vi "Imager_2.2.vi"() -> ()   [LabVIEW 2015]
doc: "You can repeat commands using for loop or while loop structures. This example shows how to use a for loop to replace the five <code>Move Relative -10000</code> commands in the previous example.\nNote that the error line needs to use a shift register in the loop, so that an error will get carried forward through later iterations.\nNow that you've seen two, here are some features common to most of our examples:\n* Place error and COM port wires in a straight line across the bottom. This is the main data flow of the diagram.\n* Start with Initialize to set timeouts and other things, and end with Close. If you don't use Close, Labview won't complain but other applications won't be able to use the COM port."
uses:
  <vilib>/Utility/config.llb/Write Key (I32).vi
  <vilib>/Utility/config.llb/Write Key (Path).vi
  <vilib>/Utility/config.llb/Write Key (String).vi
  <vilib>/Utility/config.llb/Write Key (U32).vi
  <vilib>/Utility/config.llb/Read Key (I32).vi
  <vilib>/Utility/config.llb/Read Key (Path).vi
  <vilib>/Utility/config.llb/Read Key (String).vi
  <vilib>/Utility/config.llb/NI_LVConfig.lvlib
panel:
  in  "Return home":bool
  in  "Reset Home":bool
  out "Move completed":bool
  out "Progress":string="\r\n"
  out "Image 2":T1(plugin-control)
  out "Current Plate 2":dbl
  in  "Plate Diameter (steps) 2":i32=5000
  in  "Live":bool
  in  "start path for config files":path=path "C:/images" caption="start path"
  in  "Load Settings":bool
  in  "Settings":bool
  in  "Offset to Plate 1 (steps)":i32=4000
  in  "Camera ID":u32=285941632
  in  "Pause (s)":u32
  out "Current Plate":dbl
  in  "Total Number of plates":i32=14 min=2
  out "plate number":i32
  out "Next plate number":i32
  out "first plate number":dbl
  out "Run":dbl
  in  "?":bool
  in  "EXIT":bool
  in  "Clear Settings":bool
  in  "START":bool
  in  "Plate Diameter (steps)":i32=5200
  out "Pause (seconds)":u32
  in  "Save Path":path=path "C:/images"
  in  "Port":refnum<visa-resource-name>="COM3"
  # "Plate Imager V2.0"
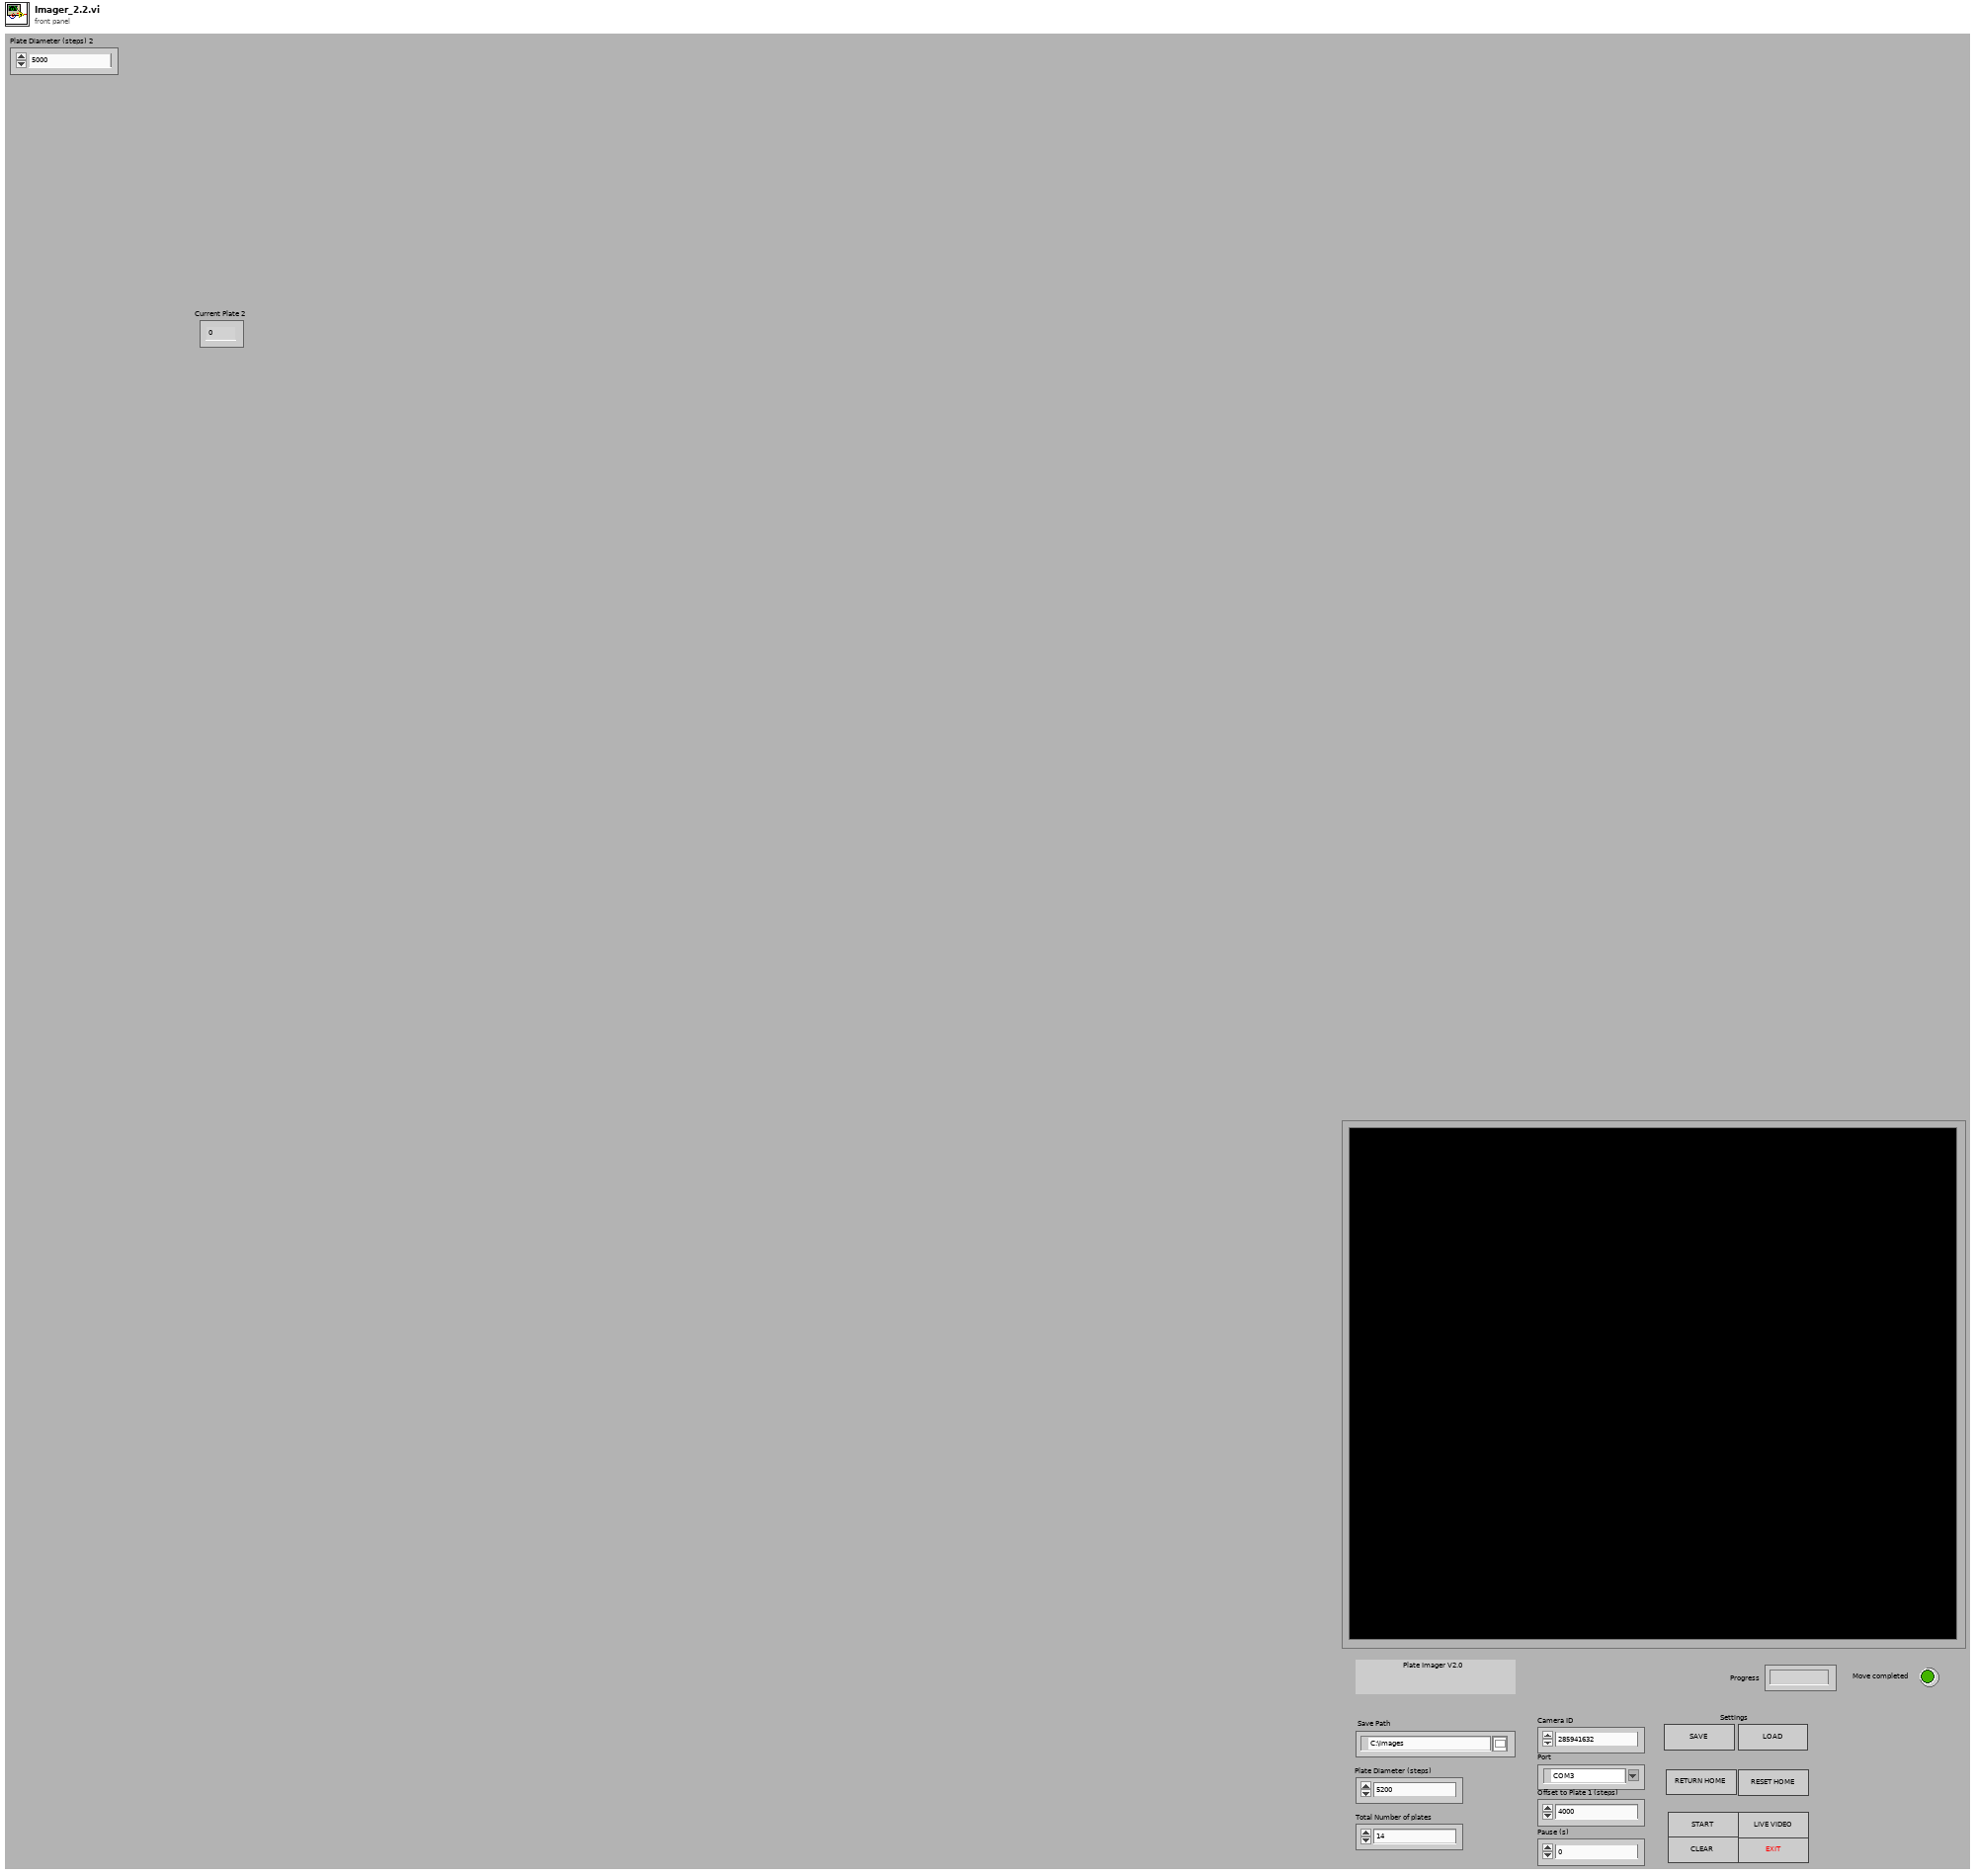
[diagram p1: front panel]
types:
  T1 = typedef "IMAQ Image.ctl" = refnum<image>
  T2 = typedef "NI_LVConfig.lvlib/Config Data RefNum.ctl" = refnum<k1>
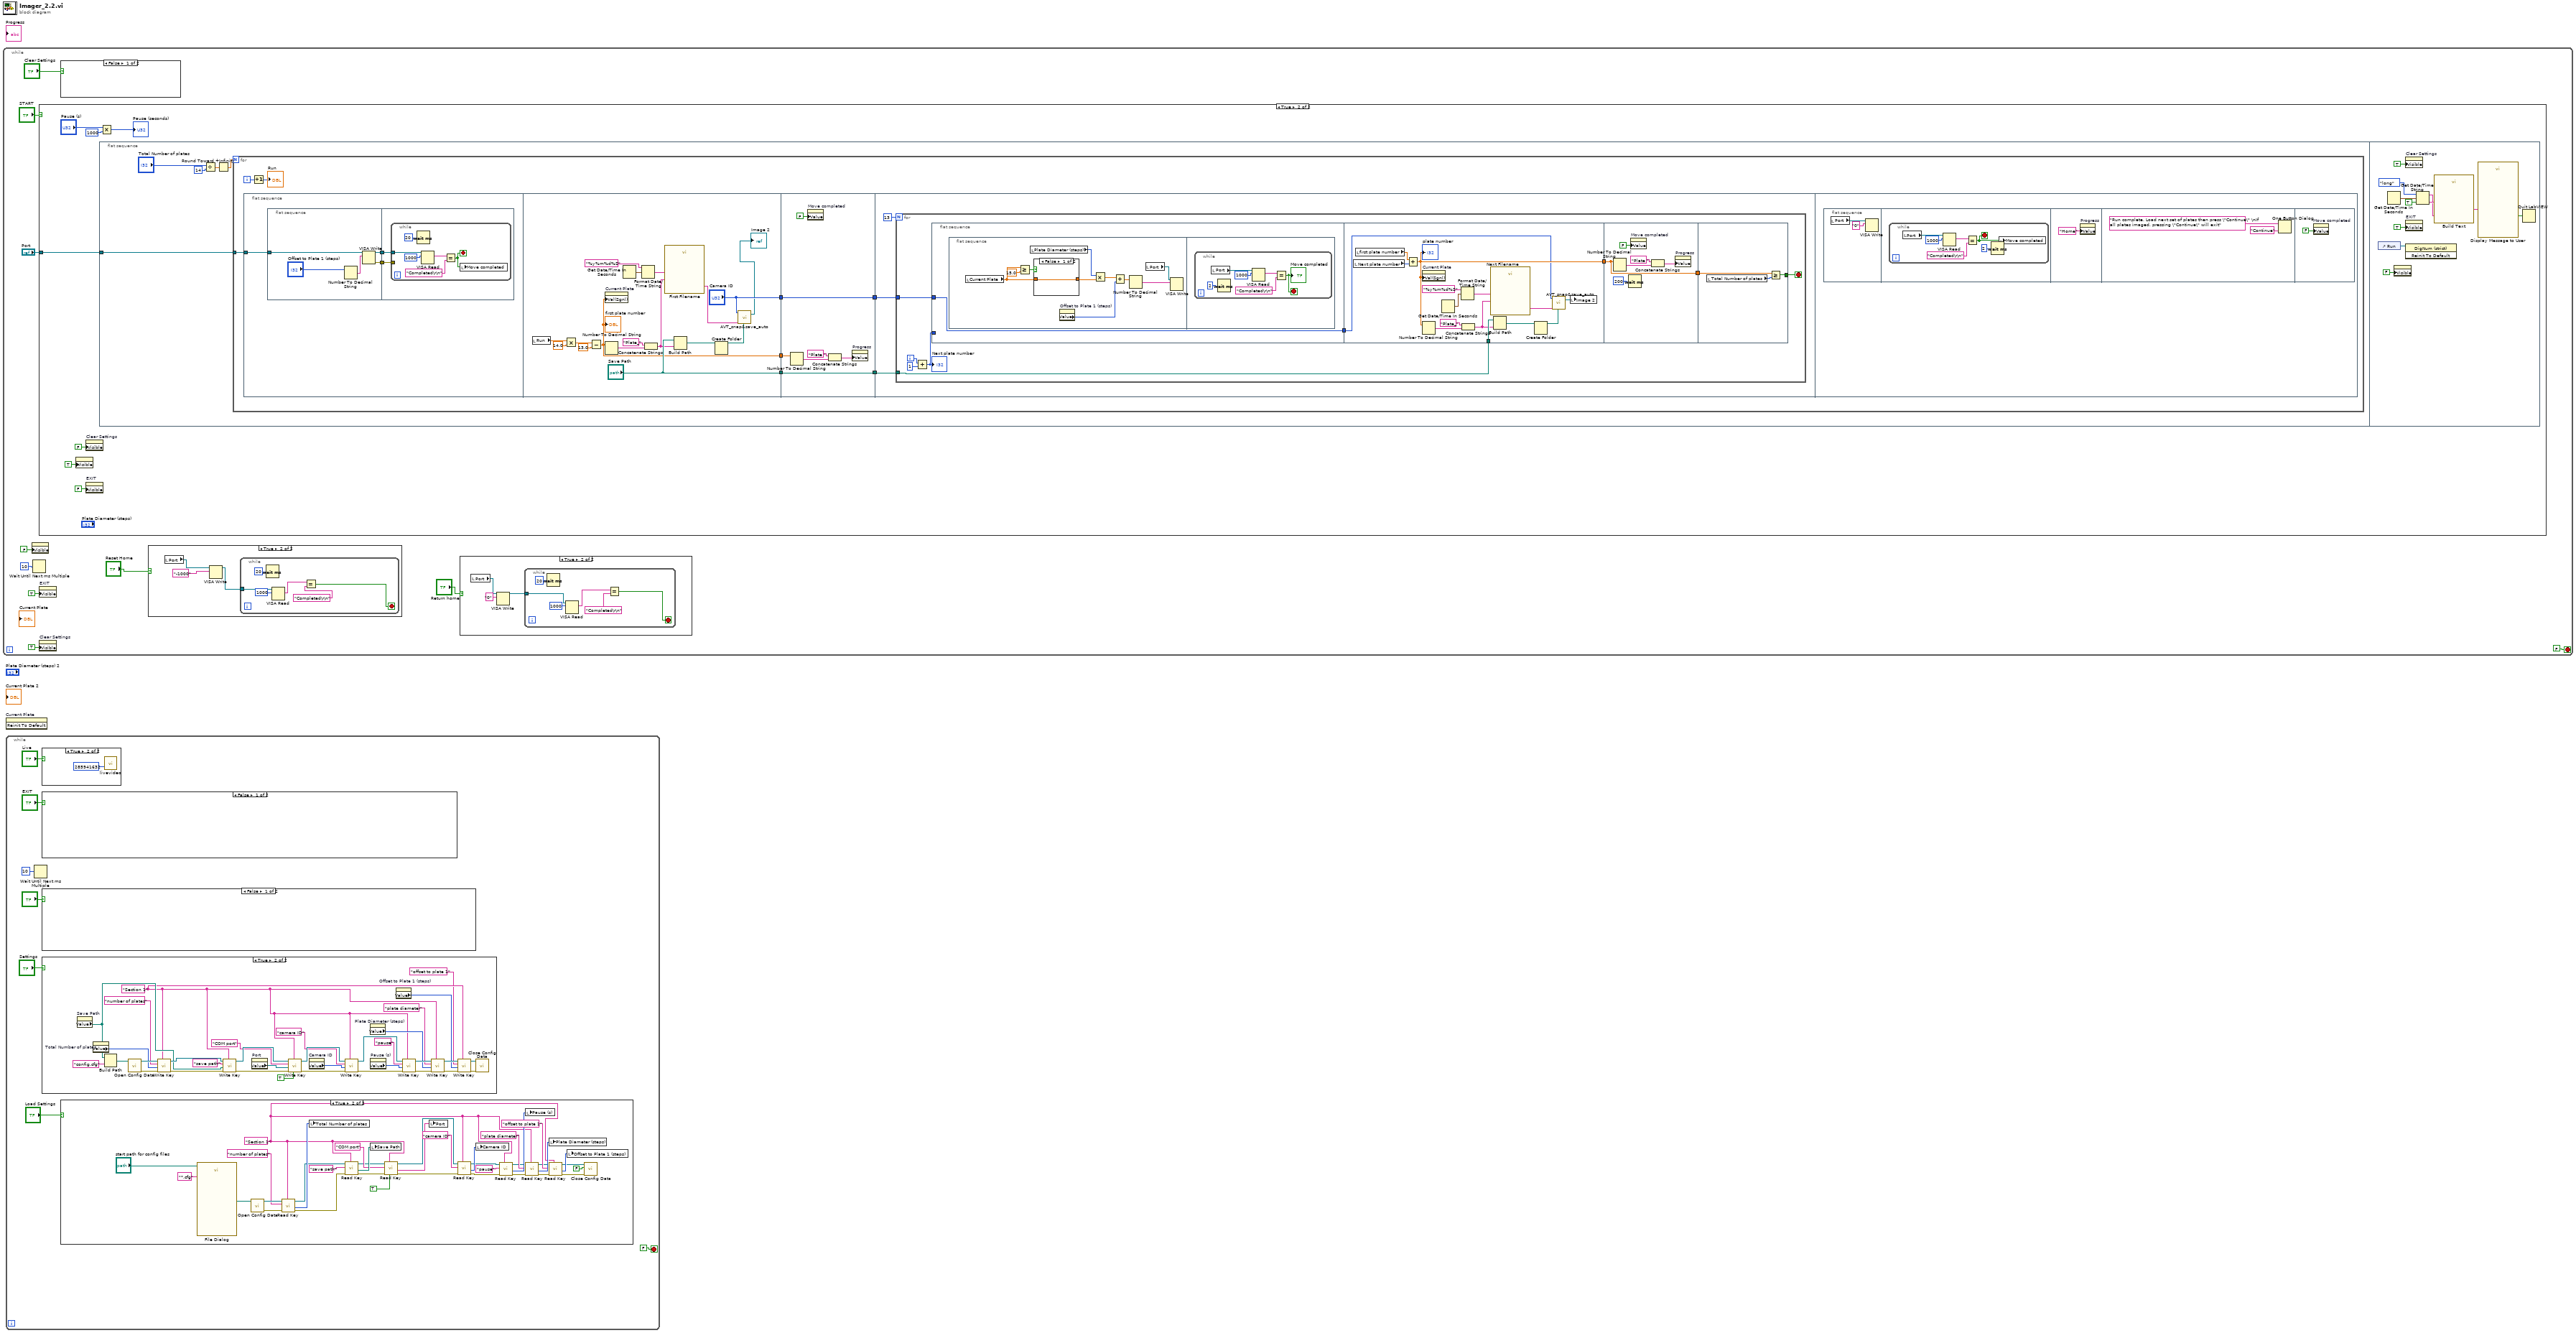
[diagram p0: block diagram]
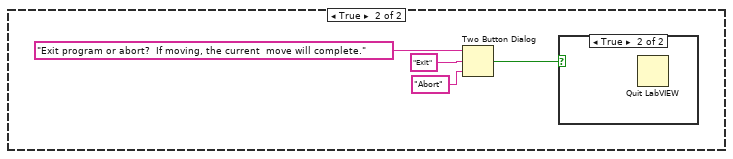
[diagram p5: hidden frame]
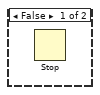
[diagram p6: hidden frame]
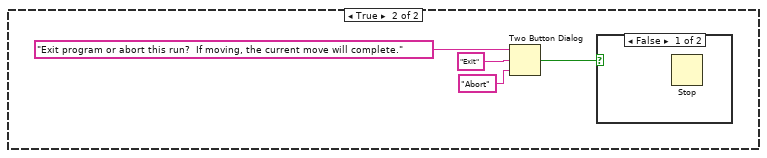
[diagram p7: hidden frame]
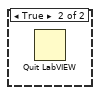
[diagram p8: hidden frame]
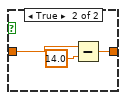
[diagram p12: hidden frame]
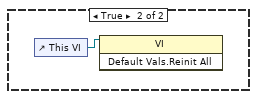
[diagram p13: hidden frame]
diagram:
  n1 = while {
    stop <- FALSE stop-if-true
    n2 = property class="Bool"("Visible"=FALSE) -> ()  [unwired: 2 in, 2 out]
    n3 = Wait Until Next ms Multiple(millisecond multiple=u32 10) -> ()  [unwired: 1 out]
    n4 = case shown="True" "START" {
      tunnel: "Port" -> [_ w29]
      frame False {
      }
      frame True {
        n5 = property class="Bool"("Visible"=TRUE) -> ()  [unwired: 2 in, 2 out]
        n6 = property on="Clear Settings" class="Bool (strict)"("Visible"=FALSE) -> ()  [unwired: 2 in, 2 out]
        n7 = property on="EXIT" class="Bool"("Visible"=FALSE) -> ()  [unwired: 2 in, 2 out]
        n8 = flat-sequence {
          tunnel: w29 -> [w36]
          frame #0 {
            n9 = Divide(x="Total Number of plates", y=14) -> (x/y=w37:dbl)
            n10 = Round Toward +Infinity(x=w37) -> (ceil(x): smallest int >= x=w38:dbl)
            n11 = for {
              N: w38 -> [_]
              tunnel: w36 -> [w46]
              i -> [w48]
              n12 = flat-sequence {
                tunnel: w46 -> [w51]
                tunnel: ["Save Path"] -> w43
                tunnel: ["Camera ID"] -> w42
                tunnel: [w66] -> w41
                tunnel: [w88] -> w45
                tunnel: [w87] -> w44
                tunnel: w41 -> [w83]
                tunnel: w42 -> [w87]
                tunnel: w43 -> [w88]
                tunnel: w45 -> [w91]
                tunnel: w44 -> [w89]
                frame #0 {
                  n13 = flat-sequence {
                    tunnel: [w56] -> w50
                    tunnel: [w55] -> w49
                    tunnel: w51 -> [w54]
                    tunnel: w50 -> [w58]
                    tunnel: w49 -> [w57]
                    frame #0 {
                      n14 = Number To Decimal String(number="Offset to Plate 1 (steps)") -> (decimal integer string=w53:string)  [unwired: 1 in]
                      n15 = VISA Write(VISA resource name=w54, write buffer=w53) -> (VISA resource name out=w56:refnum<visa-resource-name>, error out=w55:errorcluster)  [unwired: 1 in, 1 out]
                    }
                    frame #1 {
                      n16 = while {
                        tunnel: w58 -> [w64]
                        tunnel: w57 -> [_]
                        stop <- w59 stop-if-true
                        n17 = Wait (ms)(milliseconds to wait=u32 20 ("millisecond timer value")) -> ()  [unwired: 1 out]
                        n18 = VISA Read(VISA resource name=w64, byte count=u32 1000) -> (read buffer=w60:string)  [unwired: 1 in, 3 out]
                        n19 = Equal?(x=w60, y="Completed\r\n") -> (x = y?=w59:bool)
                        n20 = local write "Move completed"(w59) -> ()
                      }
                    }
                  }
                }
                frame #1 {
                  n21 = local read "Run"() -> (w79:dbl)
                  n22 = Multiply(x=w79, y=14.0) -> (x*y=w77:dbl)
                  n23 = Subtract(x=w77, y=13.0) -> (x-y=w66:dbl)
                  "first plate number" <- w66
                  n24 = property on="Current Plate" class="DigNum (strict)"("Val(Sgnl)"=w66) -> ()  [unwired: 2 in, 2 out]
                  n25 = Number To Decimal String(number=w66) -> (decimal integer string=w74:string)  [unwired: 1 in]
                  n26 = Get Date/Time In Seconds() -> (seconds since 1Jan1904=w73:timestamp)
                  n27 = Format Date/Time String(time format string (%c)="%y%m%d%S", seconds (now)=w73) -> (date/time string=w71:string)  [unwired: 1 out]
                  n28 = Concatenate Strings("Plate_" ("name or relative path"), w74) -> (w70:string)
                  n29 = call "First Filename"("time"=w71, "platenumber"=w70) -> ("Result"=w68:string)  [unwired: 2 in, 11 out]
                  n30 = Build Path(base path="Save Path", name or relative path=w70) -> (appended path=w80:path)
                  n31 = Create Folder(path (use dialog)=w80) -> (created path=w67:path)  [unwired: 1 in, 3 out]
                  n32 = call "AVT_snap&save_auto.vi"("Save Directory"=w67, "Filename"=w68, "CamID"="Camera ID") -> ("Image"=→"Image 2":T1)  [unwired: 4 in]
                }
                frame #2 {
                  n33 = Number To Decimal String(number=w83) -> (decimal integer string=w84:string)  [unwired: 1 in]
                  n34 = property on="Move completed" class="Bool (strict)"("Value"=FALSE ("Stopped")) -> ()  [unwired: 2 in, 2 out]
                  n35 = Concatenate Strings("Plate " ("Response"), w84) -> (w86:string)
                  n36 = property on="Progress" class="Str"("Value"=w86) -> ()  [unwired: 2 in, 2 out]
                }
                frame #3 {
                  n37 = for {
                    N: 13 -> [_]
                    tunnel: w91 -> [w100]
                    tunnel: w89 -> [w95]
                    i -> [w99]
                    stop <- w97 stop-if-true
                    n38 = Add(x=w99, y=1) -> (x+y=w94:i32)
                    "Next plate number" <- w94
                    n39 = flat-sequence {
                      tunnel: [w101] -> w96
                      tunnel: w95 -> [w101]
                      tunnel: w94 -> [_]
                      tunnel: w100 -> [w135]
                      tunnel: [w126] -> w93
                      tunnel: w96 -> [w125]
                      tunnel: w93 -> [w141]
                      tunnel: [w141] -> w92
                      tunnel: w92 -> [w143]
                      tunnel: [w144] -> w97
                      frame #0 {
                        n40 = flat-sequence {
                          frame #0 {
                            n41 = local read "Current Plate"() -> (w103:dbl)
                            n42 = Greater Or Equal?(x=w103, y=15.0) -> (x >= y?=w106:bool)
                            n43 = local read "Plate Diameter (steps)"() -> (w110:i32)
                            n44 = case shown="False" w106 {
                              tunnel: w103 -> [w112 w115]
                              tunnel: [w112 w113] -> w104
                              frame False {
                              }
                              frame True {
                                n45 = Subtract(x=w115, y=14.0) -> (x-y=w113:dbl)
                              }
                            }
                            n46 = property on="Offset to Plate 1 (steps)" class="DigNum (strict)"() -> ("Value"=w107:i32)  [unwired: 2 in, 2 out]
                            n47 = Multiply(x=w110, y=w104) -> (x*y=w109:dbl)
                            n48 = Add(x=w109, y=w107) -> (x+y=w108:dbl)
                            n49 = Number To Decimal String(number=w108) -> (decimal integer string=w111:string)  [unwired: 1 in]
                            n50 = local read "Port"() -> (w102:refnum<visa-resource-name>)
                            n51 = VISA Write(VISA resource name=w102, write buffer=w111) -> ()  [unwired: 1 in, 3 out]
                          }
                          frame #1 {
                            n52 = while {
                              stop <- w120 stop-if-true
                              n53 = local read "Port"() -> (w116:refnum<visa-resource-name>)
                              n54 = Wait (ms)(milliseconds to wait=u32 2 ("millisecond timer value")) -> ()  [unwired: 1 out]
                              n55 = VISA Read(VISA resource name=w116, byte count=u32 1000) -> (read buffer=w117:string)  [unwired: 1 in, 3 out]
                              n56 = Equal?(x=w117, y="Completed\r\n") -> (x = y?=w120:bool)
                              "Move completed" <- w120
                            }
                          }
                        }
                      }
                      frame #1 {
                        n57 = local read "Next plate number"() -> (w134:i32)
                        n58 = local read "first plate number"() -> (w133:dbl)
                        n59 = Add(x=w133, y=w134) -> (x+y=w126:dbl)
                        "plate number" <- w126
                        n60 = property on="Current Plate" class="DigNum (strict)"("Val(Sgnl)"=w126) -> ()  [unwired: 2 in, 2 out]
                        n61 = Number To Decimal String(number=w126) -> (decimal integer string=w131:string)  [unwired: 1 in]
                        n62 = Get Date/Time In Seconds() -> (seconds since 1Jan1904=w130:timestamp)
                        n63 = Format Date/Time String(time format string (%c)="%y%m%d%S", seconds (now)=w130) -> (date/time string=w128:string)  [unwired: 1 out]
                        n64 = Concatenate Strings("Plate_" ("string"), w131) -> (w127:string)
                        n65 = call "Next Filename"("time"=w128, "platenumber"=w127) -> ("Result"=w123:string)  [unwired: 2 in, 11 out]
                        n66 = Build Path(base path=w135, name or relative path=w127) -> (appended path=w136:path)
                        n67 = Create Folder(path (use dialog)=w136) -> (created path=w122:path)  [unwired: 1 in, 3 out]
                        n68 = call "AVT_snap&save_auto.vi"("Save Directory"=w122, "Filename"=w123, "CamID"=w125) -> ("Image"=w124:T1)  [unwired: 4 in]
                        n69 = local write "Image 2"(w124) -> ()
                      }
                      frame #2 {
                        n70 = Number To Decimal String(number=w141) -> (decimal integer string=w139:string)  [unwired: 1 in]
                        n71 = Wait (ms)(milliseconds to wait=u32 200) -> ()  [unwired: 1 out]
                        n72 = property on="Move completed" class="Bool (strict)"("Value"=FALSE ("Stopped")) -> ()  [unwired: 2 in, 2 out]
                        n73 = Concatenate Strings("Plate " ("string"), w139) -> (w138:string)
                        n74 = property on="Progress" class="Str"("Value"=w138) -> ()  [unwired: 2 in, 2 out]
                      }
                      frame #3 {
                        n75 = local read "Total Number of plates"() -> (w145:i32)
                        n76 = Greater Or Equal?(x=w143, y=w145) -> (x >= y?=w144:bool)
                      }
                    }
                  }
                }
                frame #4 {
                  n77 = flat-sequence {
                    frame #0 {
                      n78 = local read "Port"() -> (w146:refnum<visa-resource-name>)
                      n79 = VISA Write(VISA resource name=w146, write buffer="0") -> ()  [unwired: 1 in, 3 out]
                    }
                    frame #1 {
                      n80 = while {
                        stop <- w148 stop-if-true
                        n81 = local read "Port"() -> (w149:refnum<visa-resource-name>)
                        n82 = VISA Read(VISA resource name=w149, byte count=u32 1000) -> (read buffer=w150:string)  [unwired: 1 in, 3 out]
                        n83 = Equal?(x=w150, y="Completed\r\n") -> (x = y?=w148:bool)
                        n84 = Wait (ms)(milliseconds to wait=u32 2 ("millisecond timer value")) -> ()  [unwired: 1 out]
                        n85 = local write "Move completed"(w148) -> ()
                      }
                    }
                    frame #2 {
                      n86 = property on="Progress" class="Str"("Value"="Home" ("Response")) -> ()  [unwired: 2 in, 2 out]
                    }
                    frame #3 {
                      n87 = One Button Dialog(message="Run complete. Load next set of plates then press \"Continue\" \nIf all plates imaged, pressing \"Continue\" will exit", button name ("OK")="Continue") -> ()  [unwired: 1 out]
                    }
                    frame #4 {
                      n88 = property on="Move completed" class="Bool (strict)"("Value"=FALSE ("Stopped")) -> ()  [unwired: 2 in, 2 out]
                    }
                  }
                }
              }
              n89 = Increment(x=w48) -> (x+1=→"Run":i32)
            }
          }
          frame #1 {
            n90 = control-ref of="Run"() -> (w161:refnum<vi>)
            n91 = Get Date/Time In Seconds() -> (seconds since 1Jan1904=w162:timestamp)
            n92 = property class="Bool"("Visible"=FALSE) -> ()  [unwired: 2 in, 2 out]
            n93 = property on="Clear Settings" class="Bool (strict)"("Visible"=TRUE) -> ()  [unwired: 2 in, 2 out]
            n94 = property on="EXIT" class="Bool"("Visible"=TRUE) -> ()  [unwired: 2 in, 2 out]
            n95 = invoke class="DigNum (strict)" method="Reinit To Default"(reference=w161) -> ()  [unwired: 2 in, 3 out]
            n96 = Get Date/Time String(date format (0)=enum16{"short", "long", "abbreviated"}."long", seconds (now)=w162, want seconds? (F)=TRUE) -> (date string=w165:string, time string=w166:string)
            n97 = call "Build Text"("run end time"=w166, "run end date"=w165) -> ("Result"=w167:string)  [unwired: 2 in, 11 out]
            n98 = call "Display Message to User"("Message"=w167) -> ("Close Program"=w168:bool)  [unwired: 2 in, 8 out]
            n99 = Quit LabVIEW(quit? (T)=w168) -> ()
          }
        }
        n100 = Multiply(x="Pause (s)", y=u32 1000) -> (x*y=→"Pause (seconds)":u32)
      }
    }
    n101 = property on="EXIT" class="Bool"("Visible"=TRUE) -> ()  [unwired: 2 in, 2 out]
    n102 = property on="Clear Settings" class="Bool (strict)"("Visible"=TRUE) -> ()  [unwired: 2 in, 2 out]
    n103 = case shown="False" "Clear Settings" {
      frame False {
      }
      frame True {
        n104 = control-ref of="This VI"() -> (w169:refnum<vi>)
        n105 = invoke class="VI" method="Default Vals.Reinit All"(reference=w169) -> ()  [unwired: 2 in, 3 out]
      }
    }
    n106 = case shown="True" "Reset Home" {
      frame False {
      }
      frame True {
        n107 = local read "Port"() -> (w21:refnum<visa-resource-name>)
        n108 = VISA Write(VISA resource name=w21, write buffer="-1000") -> (VISA resource name out=w20:refnum<visa-resource-name>)  [unwired: 1 in, 2 out]
        n109 = while {
          tunnel: w20 -> [w27]
          stop <- w23 stop-if-true
          n110 = Wait (ms)(milliseconds to wait=u32 20) -> ()  [unwired: 1 out]
          n111 = VISA Read(VISA resource name=w27, byte count=u32 1000) -> (read buffer=w24:string)  [unwired: 1 in, 3 out]
          n112 = Equal?(x=w24, y="Completed\r\n") -> (x = y?=w23:bool)
        }
      }
    }
    n113 = case shown="True" "Return home" {
      frame False {
      }
      frame True {
        n114 = local read "Port"() -> (w13:refnum<visa-resource-name>)
        n115 = VISA Write(VISA resource name=w13, write buffer="0") -> (VISA resource name out=w11:refnum<visa-resource-name>)  [unwired: 1 in, 2 out]
        n116 = while {
          tunnel: w11 -> [w18]
          stop <- w14 stop-if-true
          n117 = Wait (ms)(milliseconds to wait=u32 20) -> ()  [unwired: 1 out]
          n118 = VISA Read(VISA resource name=w18, byte count=u32 1000) -> (read buffer=w16:string)  [unwired: 1 in, 3 out]
          n119 = Equal?(x=w16, y="Completed\r\n") -> (x = y?=w14:bool)
        }
      }
    }
  }
  n120 = invoke on="Current Plate" class="DigNum (strict)" method="Reinit To Default"() -> ()  [unwired: 3 in, 3 out]
  n121 = while {
    stop <- FALSE stop-if-true
    n122 = Wait Until Next ms Multiple(millisecond multiple=u32 10) -> ()  [unwired: 1 out]
    n123 = case shown="True" "Live" {
      frame False {
      }
      frame True {
        n124 = call "livevideo.vi"("Camera ID"=u32 285941632) -> ()  [unwired: 1 in, 1 out]
      }
    }
    n125 = case shown="False" "EXIT" {
      frame False {
      }
      frame True {
        n126 = Two Button Dialog(message="Exit program or abort?  If moving, the current  move will complete.", 1:"Abort" ("F button name (\"Cancel\")"), 2:"Exit" ("T button name (\"OK\")")) -> (T button?=w248:bool)
        n127 = case shown="True" w248 {
          frame False {
            n128 = Stop() -> ()  [unwired: 1 out]
          }
          frame True {
            n129 = Quit LabVIEW() -> ()  [unwired: 1 out]
          }
        }
      }
    }
    n130 = case shown="False" "?" {
      frame False {
      }
      frame True {
        n131 = Two Button Dialog(message="Exit program or abort this run?  If moving, the current move will complete.", 1:"Abort" ("F button name (\"Cancel\")"), 2:"Exit" ("T button name (\"OK\")")) -> (T button?=w252:bool)
        n132 = case shown="False" w252 {
          frame False {
            n133 = Stop() -> ()  [unwired: 1 out]
          }
          frame True {
            n134 = Quit LabVIEW() -> ()  [unwired: 1 out]
          }
        }
      }
    }
    n135 = case shown="True" "Settings" {
      frame False {
      }
      frame True {
        w223 = "Section 1" ("section")
        n136 = property on="Save Path" class="Path"() -> ("Value"=w236:path)  [unwired: 2 in, 2 out]
        n137 = property on="Total Number of plates" class="DigNum (strict)"() -> ("Value"=w244:i32)  [unwired: 2 in, 2 out]
        n138 = Build Path(base path=w236, name or relative path="config.cfg") -> (appended path=w246:path)
        n139 = call <vilib>:"Open Config Data.vi"("configuration file path"=w246) -> ("error out"=w239:errorcluster, "refnum"=w245:T2)  [unwired: 8 in, 1 out]
        n140 = call-poly <vilib>:"Write Key.vi"("section"=w223, "error in (no error)"=w239, "value"=w244, "key"="number of plates", "refnum"=w245) -> ("error out"=w240:errorcluster, "refnum out"=w241:T2)  [unwired: 4 in, 1 out]
        n141 = call-poly <vilib>:"Write Key.vi"("section"=w223, "error in (no error)"=w240, "value"=w236, "key"="save path", "refnum"=w241) -> ("error out"=w243:errorcluster, "refnum out"=w242:T2)  [unwired: 4 in, 1 out]
        n142 = property on="Port" class="VISAName"() -> ("Value"=w235:refnum<visa-resource-name>)  [unwired: 2 in, 2 out]
        n143 = call-poly <vilib>:"Write Key.vi"("write raw string? (F)"=TRUE, "section"=w223, "error in (no error)"=w243, "value"=w235, "key"="COM port", "refnum"=w242) -> ("error out"=w238:errorcluster, "refnum out"=w237:T2)  [unwired: 3 in, 1 out]
        n144 = property on="Camera ID" class="DigNum (strict)"() -> ("Value"=w234:u32)  [unwired: 2 in, 2 out]
        n145 = call-poly <vilib>:"Write Key.vi"("section"=w223, "error in (no error)"=w238, "value"=w234, "key"="camera ID", "refnum"=w237) -> ("error out"=w233:errorcluster, "refnum out"=w219:T2)  [unwired: 4 in, 1 out]
        n146 = property on="Plate Diameter (steps)" class="DigNum (strict)"() -> ("Value"=w229:i32)  [unwired: 2 in, 2 out]
        n147 = property on="Pause (s)" class="DigNum (strict)"() -> ("Value"=w232:u32)  [unwired: 2 in, 2 out]
        n148 = property on="Offset to Plate 1 (steps)" class="DigNum (strict)"() -> ("Value"=w224:i32)  [unwired: 2 in, 2 out]
        n149 = call-poly <vilib>:"Write Key.vi"("section"=w223, "error in (no error)"=w233, "value"=w232, "key"="pause", "refnum"=w219) -> ("error out"=w231:errorcluster, "refnum out"=w230:T2)  [unwired: 4 in, 1 out]
        n150 = call-poly <vilib>:"Write Key.vi"("section"=w223, "error in (no error)"=w231, "value"=w229, "key"="plate diameter", "refnum"=w230) -> ("error out"=w228:errorcluster, "refnum out"=w225:T2)  [unwired: 4 in, 1 out]
        n151 = call-poly <vilib>:"Write Key.vi"("section"=w223, "error in (no error)"=w228, "value"=w224, "key"="offset to plate 1", "refnum"=w225) -> ("error out"=w227:errorcluster, "refnum out"=w226:T2)  [unwired: 4 in, 1 out]
        n152 = call <vilib>:"Close Config Data.vi"("error in (no error)"=w227, "refnum"=w226) -> ()  [unwired: 8 in, 2 out]
      }
    }
    n153 = case shown="True" "Load Settings" {
      frame False {
      }
      frame True {
        w186 = "Section 1" ("section")
        n154 = call "File Dialog"("start path"="start path for config files", "pattern (all files)"="*.cfg") -> ("selected path"=w213:path)  [unwired: 10 in, 3 out]
        n155 = call <vilib>:"Open Config Data.vi"("configuration file path"=w213) -> ("error out"=w211:errorcluster, "refnum"=w212:T2)  [unwired: 8 in, 1 out]
        n156 = call-poly <vilib>:"Read Key.vi"("section"=w186, "error in (no error)"=w211, "key"="number of plates", "refnum"=w212) -> ("error out"=w206:errorcluster, "value"=w209:i32, "refnum out"=w207:T2)  [unwired: 4 in, 1 out]
        n157 = local write "Total Number of plates"(w209) -> ()
        n158 = call-poly <vilib>:"Read Key.vi"("section"=w186, "error in (no error)"=w206, "key"="save path", "refnum"=w207) -> ("error out"=w202:errorcluster, "value"=w205:path, "refnum out"=w203:T2)  [unwired: 4 in, 1 out]
        n159 = local write "Save Path"(w205) -> ()
        n160 = call-poly <vilib>:"Read Key.vi"("read raw string? (F)"=TRUE, "section"=w186, "error in (no error)"=w202, "key"="COM port", "refnum"=w203) -> ("error out"=w197:errorcluster, "value"=w201:string, "refnum out"=w198:T2)  [unwired: 3 in, 1 out]
        n161 = local write "Port"(w201) -> ()
        n162 = call-poly <vilib>:"Read Key.vi"("section"=w186, "error in (no error)"=w197, "key"="camera ID", "refnum"=w198) -> ("error out"=w194:errorcluster, "value"=w196:i32, "refnum out"=w195:T2)  [unwired: 4 in, 1 out]
        n163 = local write "Camera ID"(w196) -> ()
        n164 = call-poly <vilib>:"Read Key.vi"("section"=w186, "error in (no error)"=w194, "key"="pause", "refnum"=w195) -> ("error out"=w189:errorcluster, "value"=w192:i32, "refnum out"=w190:T2)  [unwired: 4 in, 1 out]
        n165 = local write "Pause (s)"(w192) -> ()
        n166 = call-poly <vilib>:"Read Key.vi"("section"=w186, "error in (no error)"=w189, "key"="plate diameter", "refnum"=w190) -> ("error out"=w184:errorcluster, "value"=w188:i32, "refnum out"=w185:T2)  [unwired: 4 in, 1 out]
        n167 = local write "Plate Diameter (steps)"(w188) -> ()
        n168 = call-poly <vilib>:"Read Key.vi"("section"=w186, "error in (no error)"=w184, "key"="offset to plate 1", "refnum"=w185) -> ("error out"=w182:errorcluster, "value"=w183:i32, "refnum out"=w181:T2)  [unwired: 4 in, 1 out]
        n169 = local write "Offset to Plate 1 (steps)"(w183) -> ()
        n170 = call <vilib>:"Close Config Data.vi"("error in (no error)"=w182, "write file if changed (T)"=FALSE, "refnum"=w181) -> ()  [unwired: 7 in, 2 out]
      }
    }
  }
